vi "DAQmx.Auto Configure.vi"(8 "error in (no error)":errorcluster, 11 "DAQmx in":refnum<class "DAQmx.lvclass">) -> (0 "error out":errorcluster, 1 "Configuration.Timing.Sampling":T1={"Fs"=204789.0, "#s"=15753} {"Fs" format="%#_13g"}, 2 "Devices":T10[](array[typedef]), 3 "DAQmx out":refnum<class "DAQmx.lvclass">, 4 "Configuration.AO":T2 {"output terminal configuration" items=[""=-1, "Differential"=10106, "Pseudodifferential"=12529]}, 6 "Configuration.AI":T6 {"input terminal configuration" items=[""=-1, "Differential"=10106, "Pseudodifferential"=12529]; "Coupling" items=[""=0, "AC"=10045, "DC"=10050, "GND"=10066]})   [LabVIEW 2019, in "DAQmx.lvclass"]
uses:
  DAQmx.lvclass
  typedefs/DeviceInfo--Cluster.ctl
  typedefs/DAQ.Config.AI--Cluster--Array.ctl
  typedefs/DAQ.Config.AI--Cluster.ctl
  typedefs/DAQ.Config.AI.Coupling--enum.ctl
  typedefs/DAQ.Config.AI.Range--enum.ctl
  typedefs/DAQ.Config.Device Type--enum.ctl
  typedefs/DAQ.Config.AO--Cluster--Array.ctl
  typedefs/DAQ.Config.AO--Cluster.ctl
  typedefs/DAQ.Config.AO.Range--enum.ctl
  typedefs/DAQ.Config.Timing.Sampling--Cluster.ctl
  DAQmx.lvclass/DAQmx.ctl
  <resource>/objmgr/daqmx.rc
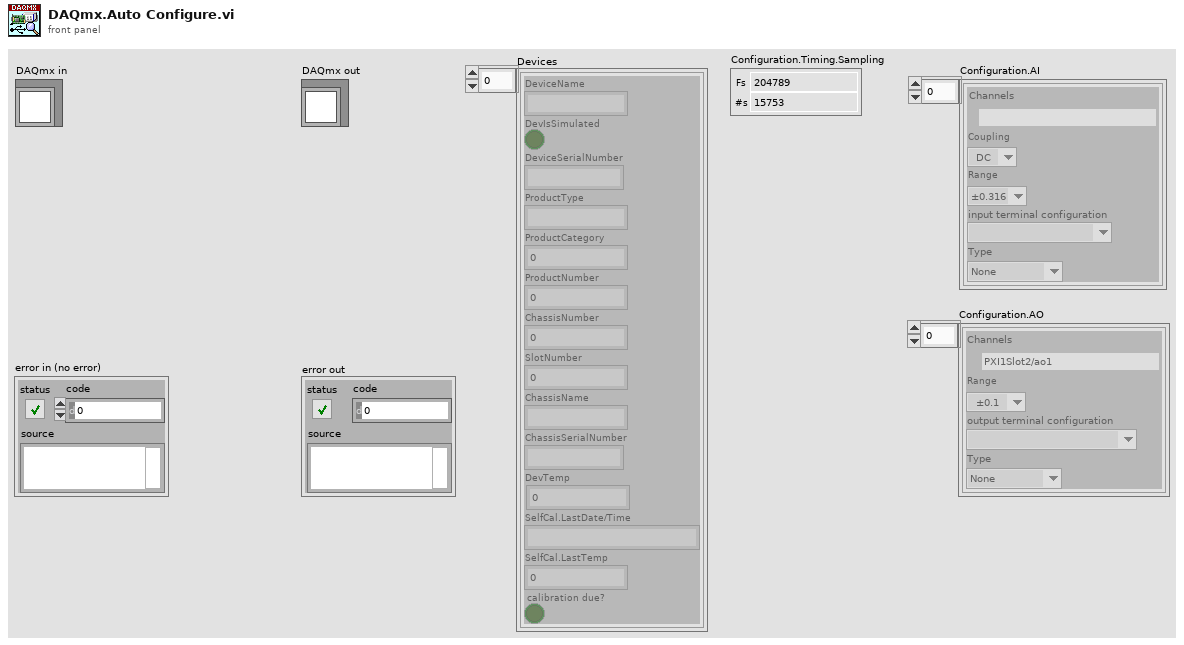
[diagram p1: front panel]
types:
  T1 = typedef "DAQmx.lvclass/DAQ.Config.Timing.Sampling--Cluster.ctl" = cluster{"Fs":dbl, "#s":i32}
  T2 = typedef "DAQmx.lvclass/DAQ.Config.AO--Cluster--Array.ctl" = T3[]
  T3 = typedef "DAQmx.lvclass/DAQ.Config.AO--Cluster.ctl" = cluster{"Channels":tag, "Range":T4, "output terminal configuration":i32, "Type":T5}
  T4 = typedef "DAQmx.lvclass/DAQ.Config.AO.Range--enum.ctl" = enum16{"±0.1", "±1.0", "±3.5", "±10.0", ""}
  T5 = typedef "DAQmx.lvclass/DAQ.Config.Device Type--enum.ctl" = enum16{"None", "USB-4431", "PXI-446x"}
  T6 = typedef "DAQmx.lvclass/DAQ.Config.AI--Cluster--Array.ctl" = T7[]
  T7 = typedef "DAQmx.lvclass/DAQ.Config.AI--Cluster.ctl" = cluster{"Channels":tag, "Coupling":T8, "Range":T9, "input terminal configuration":i32, "Type":T5}
  T8 = typedef "DAQmx.lvclass/DAQ.Config.AI.Coupling--enum.ctl" = u16
  T9 = typedef "DAQmx.lvclass/DAQ.Config.AI.Range--enum.ctl" = enum16{"±0.316", "±1.00", "±3.16", "±10.0", "±31.6", "±42.4", ""}
  T10 = typedef "DAQmx.lvclass/DeviceInfo--Cluster.ctl" = cluster{"DeviceName":string, "DevIsSimulated":bool, "DeviceSerialNumber":string, "ProductType":string, "ProductCategory":i32, "ProductNumber":u32, "ChassisNumber":u32, "SlotNumber":u32, "ChassisName":string, "ChassisSerialNumber":string, "DevTemp":dbl, "SelfCal.LastDate/Time":string, "SelfCal.LastTemp":dbl, "calibration due?":bool}
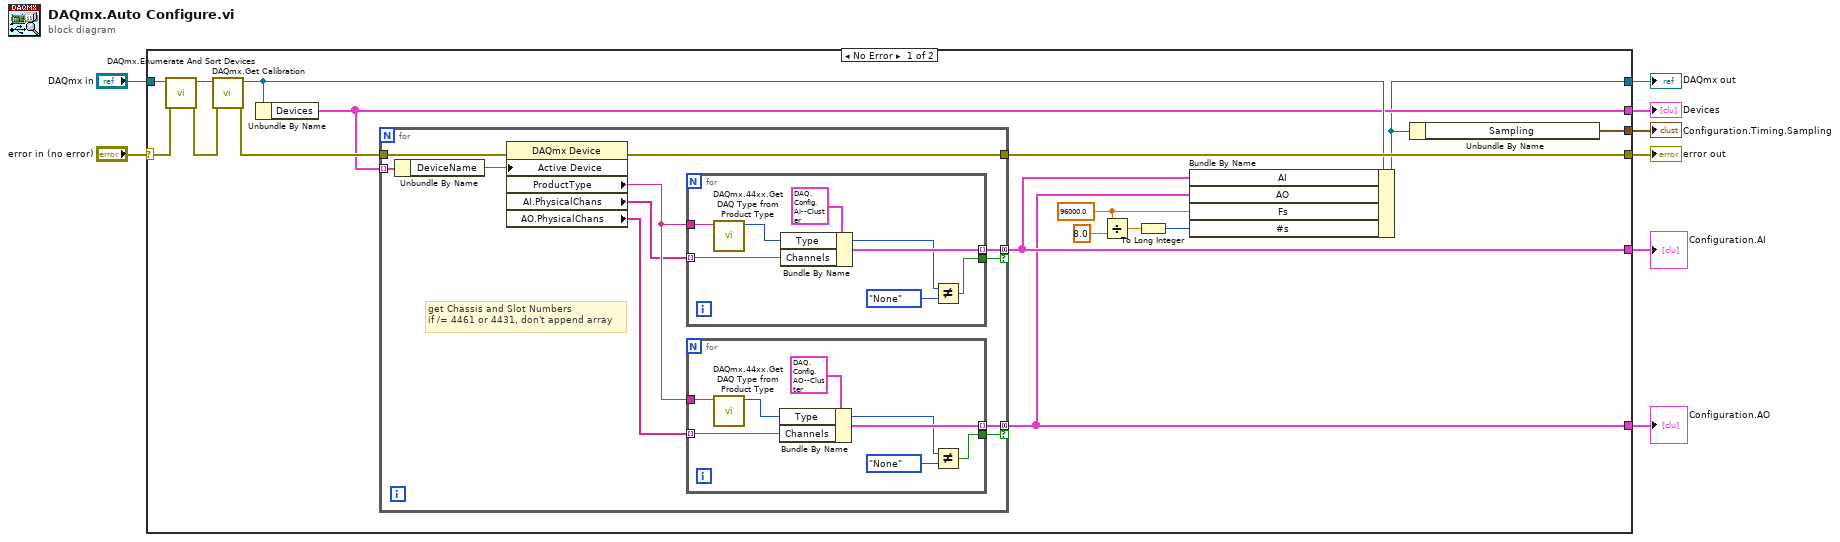
[diagram p0: block diagram]
diagram:
  n1 = case shown="No Error" "error in (no error)" {
    selector: "error in (no error)" -> [w22 w50]
    tunnel: [w24 w50] -> w8
    tunnel: "DAQmx in" -> [w23 w51]
    tunnel: [w10 w51] -> w6
    tunnel: [w15 _] -> w4
    tunnel: [w21 _] -> w3
    tunnel: [w20 _] -> w2
    tunnel: [w9 _] -> w1
    frame No Error {
      w14 = 96000.0 ("AI.Min")
      n2 = call "DAQmx.Enumerate And Sort Devices.vi"("error in (no error)"=w22, "DAQmx in"=w23) -> ("error out"=w18:errorcluster, "DAQmx out"=w19:refnum<class "DAQmx.lvclass">)  [unwired: 7 in, 1 out]
      n3 = call "DAQmx.Get Calibration.vi"("error in (no error)"=w18, "DAQmx in"=w19) -> ("error out"=w17:errorcluster, "DAQmx out"=w16:refnum<class "DAQmx.lvclass">)  [unwired: 7 in, 1 out]
      n4 = Unbundle By Name(w16) -> ("Devices"=w15:T10[])
      n5 = for {
        tunnel: [w27] -> w24
        tunnel: [w35] -> w21 mode=concatenating if=w34
        tunnel: w17 -> [w33]
        tunnel: w15 -> [w32] mode=indexing
        tunnel: [w29] -> w20 mode=concatenating if=w28
        # "get Chassis and Slot Numbers\nif /= 4461 or 4431, don't append array"
        n6 = Unbundle By Name(w32) -> ("DeviceName"=w31:string)
        n7 = property class="DAQmx Device"(error in=w33, "Active Device"=w31) -> (error out=w27:errorcluster, "ProductType"=w30:string, "AI.PhysicalChans"=w25:tag[], "AO.PhysicalChans"=w26:tag[])  [unwired: 1 in, 1 out]
        n8 = for {
          tunnel: [w42] -> w35 mode=indexing
          tunnel: w30 -> [w38]
          tunnel: [w37] -> w34
          tunnel: w25 -> [w39] mode=indexing
          n9 = call "DAQmx.44xx.Get DAQ Type from Product Type.vi"("ProductType"=w38) -> ("DAQ Type"=w36:T5)  [unwired: 10 in]
          n10 = Bundle By Name(cluster=T7 {"Channels"="PXI1Slot2/ai0", "Coupling"=10050, "Range"=enum."±0.316", "input terminal configuration"=-1, "Type"=enum."PXI-446x"} ("AI.Config"), "Type"=w36, "Channels"=w39) -> (w42:T7)
          n11 = Not Equal?(x=w36, y=DAQ.Config.Device_Type--enum."None") -> (x != y?=w37:bool)
        }
        n12 = for {
          tunnel: [w45] -> w29 mode=indexing
          tunnel: w30 -> [w49]
          tunnel: [w44] -> w28
          tunnel: w26 -> [w47] mode=indexing
          n13 = call "DAQmx.44xx.Get DAQ Type from Product Type.vi"("ProductType"=w49) -> ("DAQ Type"=w43:T5)  [unwired: 10 in]
          n14 = Bundle By Name(cluster=T3 {"Channels"="PXI1Slot2/ao1", "Range"=enum."±0.1", "output terminal configuration"=-1, "Type"=enum."USB-4431"} ("AO.config"), "Type"=w43, "Channels"=w47) -> (w45:T3)
          n15 = Not Equal?(x=w43, y=DAQ.Config.Device_Type--enum."None") -> (x != y?=w44:bool)
        }
      }
      n16 = Divide(x=w14, y=8.0) -> (x/y=w12:dbl)
      n17 = To Long Integer(number=w12) -> (32bit integer=w11:i32)
      n18 = Bundle By Name(cluster=w16, "AI"=w21, "AO"=w20, "Fs"=w14, "#s"=w11) -> (w10:refnum<class "DAQmx.lvclass">)
      n19 = Unbundle By Name(w10) -> ("Sampling"=w9:T1)
    }
    frame Error {
    }
  }
  "error out" <- w8
  "DAQmx out" <- w6
  "Devices" <- w4
  "Configuration.AI" <- w3
  "Configuration.AO" <- w2
  "Configuration.Timing.Sampling" <- w1
